vi "set time on rio.vi"() -> ()   [LabVIEW 2015]
uses:
  <vilib>/nisyscfg/nisyscfg.lvlib
  <vilib>/nisyscfg/Save Changes (System).vi
  <vilib>/nisyscfg/Close (System).vi
panel:
  out "number: 0 to 1":dbl
  out "x+1":dbl
  out "Numeric":i32
  out "Detailed Result 2":string caption="Detailed Result"
  out "Wait Until Complete (T)":bool=TRUE
  out "error out":errorcluster
  out "Detailed Result":string
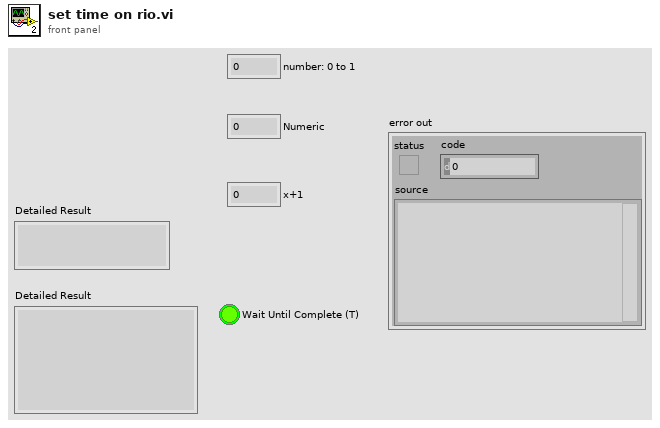
[diagram p1: front panel]
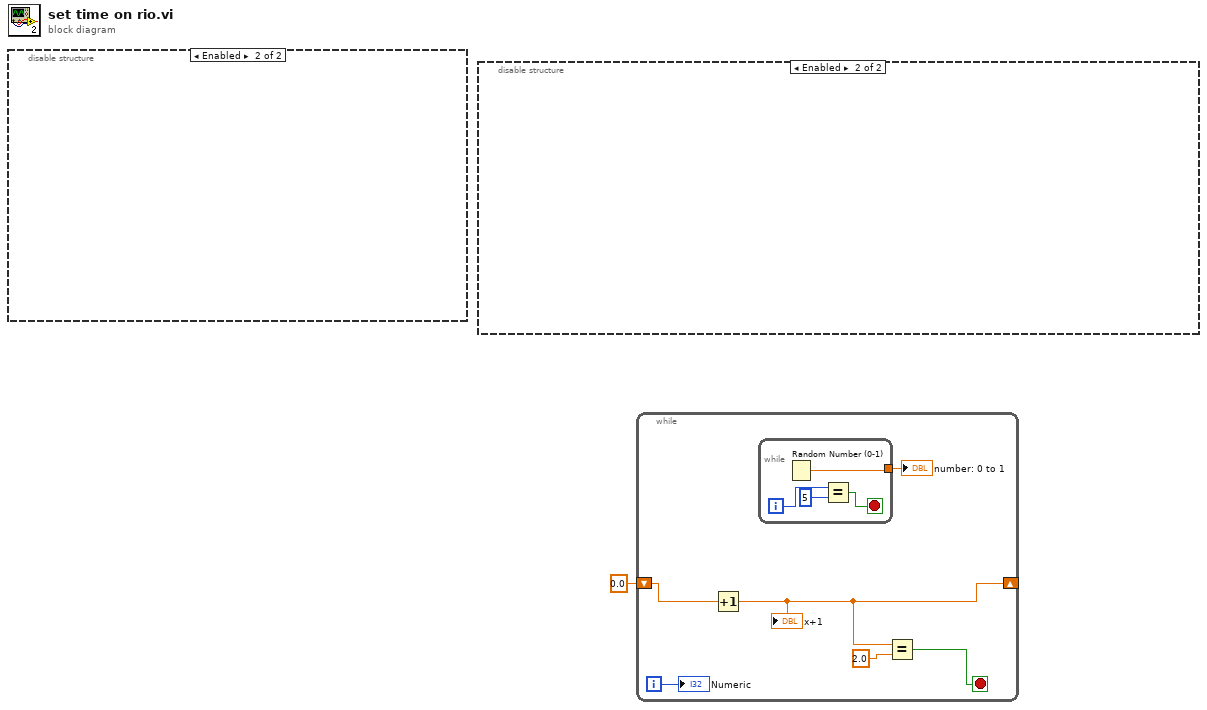
[diagram p0: block diagram]
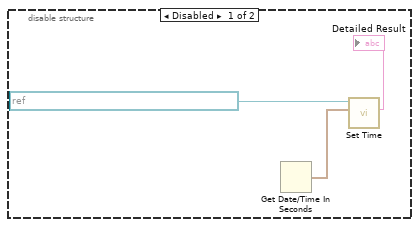
[diagram p2: hidden frame]
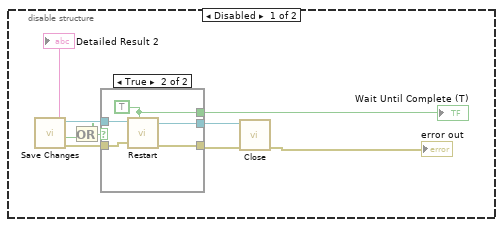
[diagram p3: hidden frame]
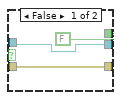
[diagram p4: hidden frame]
diagram:
  n1 = disable-structure shown="Enabled" {
    frame Disabled {
      n2 = Get Date/Time In Seconds() -> (seconds since 1Jan1904=w4:timestamp)
      n3 = call <vilib>:"Set Time.vi"("Time"=w4, "Session in (localhost)"=refnum<k21> "NI-sbRIO9636-01A93195 (192.168.1.99)" ("System Configuration")) -> ("Detailed Result"=→"Detailed Result":string)  [unwired: 6 in, 3 out]
    }
    frame Enabled {
    }
  }
  n4 = disable-structure shown="Enabled" {
    frame Disabled {
      n5 = call-poly <vilib>:"Save Changes.vi"() -> ("error out"=w13:errorcluster, "Changes Require Restart"=w10:bool, "Detailed Result"=→"Detailed Result 2":string, "Session out"=w14:refnum<k21>)  [unwired: 8 in]
      n6 = Or(y=w10) -> (x=w9:bool, x .or. y?=w5:bool)
      n7 = case shown="True" w5 {
        tunnel: w14 -> [w15 w22]
        tunnel: w13 -> [w16 w21]
        tunnel: [w16 w20] -> w7
        tunnel: [FALSE ("Wait Until Complete (T)") w19] -> w12
        tunnel: [w15 w18] -> w8
        frame False {
        }
        frame True {
          w19 = TRUE ("Wait Until Complete (T)")
          n8 = call <vilib>:"Restart.vi"("Wait Until Complete (T)"=w19, "error in (no error)"=w21, "Session in"=w22) -> ("error out"=w20:errorcluster, "Session out"=w18:refnum<k21>)  [unwired: 6 in, 1 out]
        }
      }
      "Wait Until Complete (T)" <- w12
      n9 = call-poly <vilib>:"Close.vi"("error in (no error)"=w7, "Session in"=w8) -> ("error out"=→"error out":errorcluster)  [unwired: 9 in]
    }
    frame Enabled {
    }
  }
  n10 = while {
    shift-right: [w25] -> _
    shift-left: 0.0 -> [w27]
    i -> [w28]
    stop <- w26 stop-if-true
    n11 = Increment(x=w27) -> (x+1=w25:dbl)
    "x+1" <- w25
    n12 = while {
      tunnel: [w32] -> w23
      i -> [w30]
      stop <- w31 stop-if-true
      n13 = Random Number (0-1)() -> (number: 0 to 1=w32:dbl)
      n14 = Equal?(x=w30, y=5) -> (x = y?=w31:bool)
    }
    "number: 0 to 1" <- w23
    n15 = Equal?(x=w25, y=2.0) -> (x = y?=w26:bool)
    "Numeric" <- w28
  }
